vi "Modules Page.vi"(8 "error in (no error)":errorcluster, 11 "Node Ptr":T2 format="%.0x") -> (0 "error out":errorcluster)   [LabVIEW 2017, in "Routing and Faulting System Explorer.lvlib"]
uses:
  Routing and Faulting System Explorer.lvlib
  <vilib>/NI Veristand/Custom Device API/Custom Device Item Ref.ctl
  Module Row.ctl
  Modules Page Controls.ctl
  <vilib>/NI Veristand/Custom Device API/Custom Device API.lvlib
  Scripting/Routing and Faulting Scripting.lvlib
  Shared/UI Common/UI Common.lvlib
panel:
  in  "Modules":T1[](array[typedef])
  in  "SHDocVw.IWebBrowser":refnum<k7>(container)
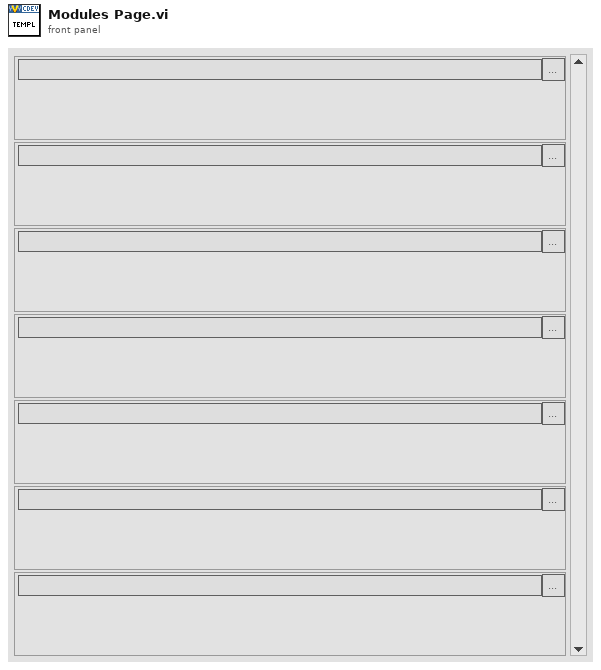
[diagram p1: front panel]
types:
  T1 = typedef "Routing and Faulting System Explorer.lvlib/Module Row.ctl" = cluster{"Module path":string, "Edit":bool, "Description":string}
  T2 = typedef "Custom Device API.lvlib/Custom Device Item Ref.ctl" = u64
  T3 = typedef "Routing and Faulting System Explorer.lvlib/Modules Page Controls.ctl" = cluster{"Modules":refnum<vi>}
  T4 = typedef "Custom Device API.lvlib/Custom Device Commands.ctl" = enum16{"Default", "Item renamed", "Shutdown", "Dynamic button pressed"}
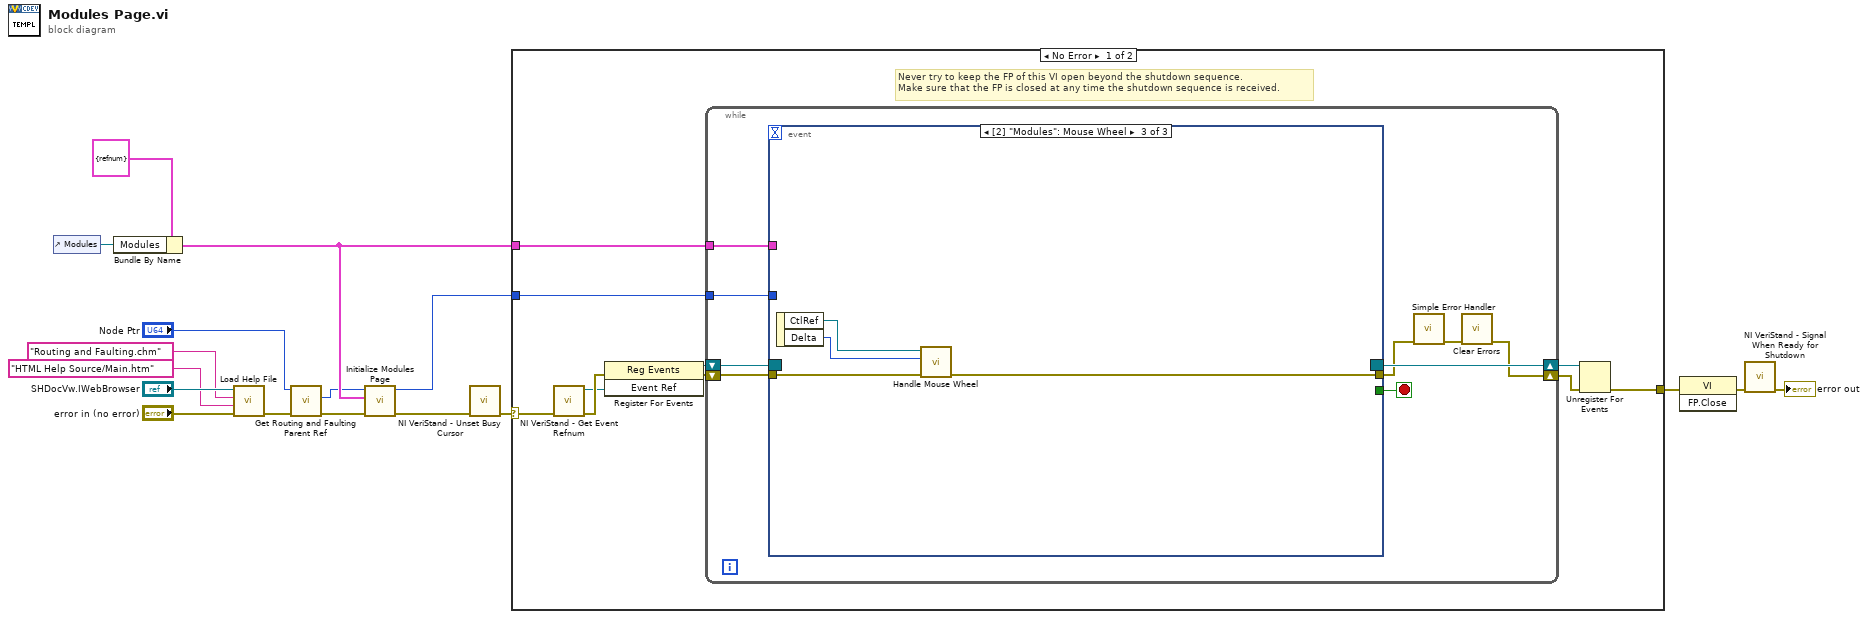
[diagram p0: block diagram]
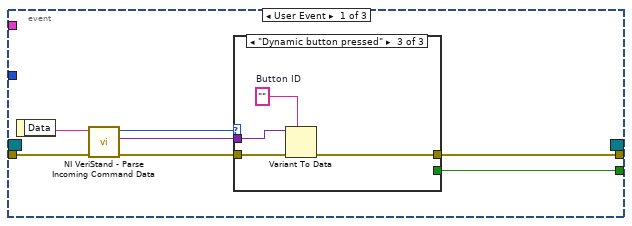
[diagram p2: hidden frame]
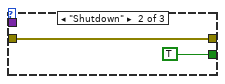
[diagram p4: hidden frame]
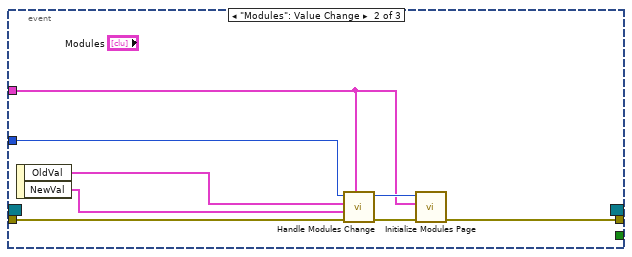
[diagram p5: hidden frame]
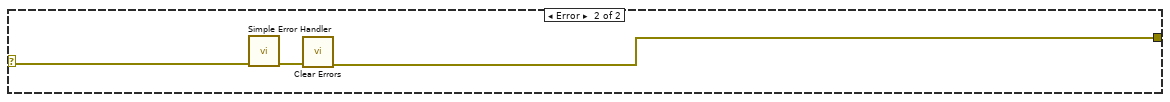
[diagram p6: hidden frame]
diagram:
  n1 = control-ref of="Modules"() -> (w7:refnum<vi>)
  n2 = Bundle By Name(cluster=T3 {"Modules"=refnum} ("Modules Page Controls"), "Modules"=w7) -> (w6:T3)
  n3 = call "Load Help File.vi"("error in (no error)"="error in (no error)", "HTML File to Load"="HTML Help Source/Main.htm" ("HTML File"), "Main CHM File"="Routing and Faulting.chm" ("CD_CHM_FileName"), "Browser"="SHDocVw.IWebBrowser") -> ("error out"=w5:errorcluster)  [unwired: 7 in]
  n4 = call "Get Routing and Faulting Parent Ref.vi"("error in (no error)"=w5, "Routing and Faulting Child Ref in"="Node Ptr") -> ("error out"=w4:errorcluster, "Routing and Faulting Ref out"=w2:T2)  [unwired: 7 in, 1 out]
  n5 = call "Initialize Modules Page.vi"("error in (no error)"=w4, "Modules Page Controls"=w6, "Routing and Faulting Ref in"=w2) -> ("error out"=w9:errorcluster, "Routing and Faulting Ref out"=w1:T2)  [unwired: 7 in]
  n6 = call <vilib>:"NI VeriStand - Unset Busy Cursor.vi"("error in (no error)"=w9) -> ("error out"=w14:errorcluster)  [unwired: 10 out]
  n7 = case shown="No Error" w14 {
    selector: w14 -> [w20 w65]
    tunnel: [w24 w63] -> w17
    tunnel: w6 -> [w19 _]
    tunnel: w1 -> [w18 _]
    frame No Error {
      # "Never try to keep the FP of this VI open beyond the shutdown sequence.\nMake sure that the FP is closed at any time the shutdown sequence is received."
      n8 = call <vilib>:"NI VeriStand - Get Event Refnum.vi"("error in (no error)"=w20) -> ("error out"=w27:errorcluster, "Event Ref"=w23:refnum<user-event>)  [unwired: 9 out]
      n9 = register-events(error in=w27, w23) -> (reference out=w21:refnum<event-registration>, error out=w22:errorcluster)  [unwired: 1 in]
      n10 = while {
        shift-right: [w30] -> w25
        shift-left: w22 -> [w35]
        shift-right: [w36] -> w26
        shift-left: w21 -> [w34]
        tunnel: w19 -> [w29]
        tunnel: w18 -> [w28]
        stop <- w33 stop-if-true
        n11 = event shown="[2] \"Modules\": Mouse Wheel" {
          selector: w34 -> [_ _ _]
          dyn-events: [_ _ _] -> w36
          timeout: _ -> [_ _ _]
          tunnel: w35 -> [w43 w56 w62]
          tunnel: [w39 _ _] -> w33
          tunnel: [w38 w51 w61] -> w32
          tunnel: w29 -> [_ w52 _]
          tunnel: w28 -> [_ w55 _]
          event User Event {
            n12 = event-data() -> ("Data"=w42:string)  [unwired: 1 out]
            n13 = call <vilib>:"NI VeriStand - Parse Incoming Command Data.vi"("error in (no error)"=w43, "Incoming data"=w42) -> ("error out"=w41:errorcluster, "Outgoing data"=w37:variant, "Action"=w40:T4)  [unwired: 7 out]
            n14 = case shown="\"Dynamic button pressed\"" w40 {
              tunnel: w41 -> [w44 w45 w50]
              tunnel: [_ TRUE _] -> w39
              tunnel: [w44 w45 w47] -> w38
              tunnel: w37 -> [_ _ w49]
              frame "Default", Default {
              }
              frame "Shutdown" {
              }
              frame "Dynamic button pressed" {
                w48 = ""  # Button ID
                n15 = Variant To Data(error in=w50, type=w48, Variant=w49) -> (error out=w47:errorcluster)  [unwired: 1 out]
              }
            }
          }
          event "Modules": Value Change {
            n16 = event-data() -> ("OldVal"=w58:T1[], "NewVal"=w57:T1[])  [unwired: 1 out]
            n17 = call "Handle Modules Change.vi"("Modules Page Controls"=w52, "error in (no error)"=w56, "NewVal"=w57, "OldVal"=w58, "Routing and Faulting Ref in"=w55) -> ("error out"=w54:errorcluster, "Routing and Faulting Ref out"=w53:T2)  [unwired: 5 in]
            n18 = call "Initialize Modules Page.vi"("error in (no error)"=w54, "Modules Page Controls"=w52, "Routing and Faulting Ref in"=w53) -> ("error out"=w51:errorcluster)  [unwired: 7 in, 1 out]
          }
          event "Modules": Mouse Wheel {
            n19 = event-data() -> ("CtlRef"=w60:refnum<vi>, "Delta"=w59:i32)  [unwired: 1 out]
            n20 = call "Handle Mouse Wheel.vi"("error in (no error)"=w62, "delta"=w59, "Array Refnum"=w60) -> ("error out"=w61:errorcluster)  [unwired: 7 in, 1 out]
          }
        }
        n21 = call <vilib>:"Simple Error Handler.vi"("error in (no error)"=w32) -> ("error out"=w31:errorcluster)  [unwired: 1 in, 7 out]
        n22 = call <vilib>:"Clear Errors.vi"("error in (no error)"=w31) -> ("error out"=w30:errorcluster)  [unwired: 1 in, 5 out]
      }
      n23 = Unregister For Events(event registration refnum=w26, error in=w25) -> (error out=w24:errorcluster)
    }
    frame Error {
      n24 = call <vilib>:"Simple Error Handler.vi"("error in (no error)"=w65) -> ("error out"=w64:errorcluster)  [unwired: 1 in, 7 out]
      n25 = call <vilib>:"Clear Errors.vi"("error in (no error)"=w64) -> ("error out"=w63:errorcluster)  [unwired: 1 in, 5 out]
    }
  }
  n26 = invoke class="VI" method="FP.Close"(error in=w17) -> (error out=w16:errorcluster)  [unwired: 2 in, 2 out]
  n27 = call <vilib>:"NI VeriStand - Signal When Ready for Shutdown.vi"("error in (no error)"=w16) -> ("error out"=→"error out":errorcluster)  [unwired: 10 out]
